vi "Status.vi"() -> ()   [LabVIEW 2013]
panel:
  out "Wait for instruction...":string="Wait for instruction..."
  out "Reading...":string="Reading..."
  out "Abort":string="Abort"
  out "Positon Set":string="Positon Set"
  out "IDLE":string="IDLE"
  out "Disconnected":string="Disconnected"
  out "Connected":string="Connected"
  out "Work in progress...":string="Work in progress..."
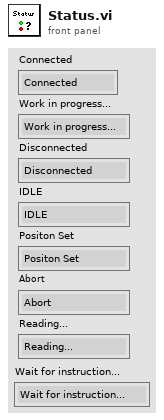
[diagram p1: front panel]
diagram:
